vi "Dynamic_call_speed_test.vi"() -> ()   [LabVIEW 2010]
uses:
  Gen Trav/Traverse_cluster.ctl
  Gen Trav/Spacing.ctl
  Controls/Multi_run_mode.ctl
  Globals/Constants_global.vi
panel:
  out "Time taken in seconds":dbl
  out "Error Messages":string
  in  "Traverse line":T1={"Start X"=0.0, "Start Y"=0.0, "Start Z"=0.0, "End X"=0.0, "End Y"=0.0, "End Z"=0.0, "No. of pts."=0, "Spacing"=enum."Linear", "Filename"=path "", "Tunnel Speed"=0.0, "Averaging time (min)"=0.0, "Extra Commands"="", "Specific Arguments"=";2", "Emission Rate (l/min)"=0.0, "Trace Gas Concentration (%)"=0.0, "Density Ratio"="", "Comments"="", "Row No"=0, "Row Type Selector"=enum."Run VI Named:", "Completion time"="", "Row Duration (mins)"=0.0, "No. of Valid pts."=0, "Meas Setup File"=""} {"Row Duration (mins)" format="%#.1f"; "Row No" min=0; "Trace Gas Concentration (%)" min=0.0 format="%#.2f"; "Emission Rate (l/min)" format="%#.2f"; "Tunnel Speed" format="%#.2f"; "Start X" format="%#.2f"; "Start Y" format="%#.2f"; "Start Z" format="%#.2f"; "End X" format="%#.2f"; "End Y" format="%#.2f"; "End Z" format="%#.2f"; "Averaging time (min)" min=0.0 format="%#.1f"}
  in  "Number of calls":i32
  # "X           Y            Z"
  # "Start"
  # "End"
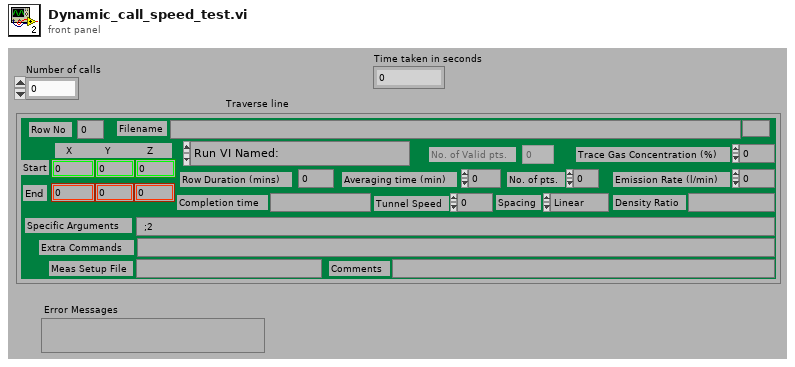
[diagram p1: front panel]
types:
  T1 = typedef "Traverse_cluster.ctl" = cluster{"Start X":dbl, "Start Y":dbl, "Start Z":dbl, "End X":dbl, "End Y":dbl, "End Z":dbl, "No. of pts.":i32, "Spacing":T2, "Filename":path, "Tunnel Speed":dbl, "Averaging time (min)":dbl, "Extra Commands":string, "Specific Arguments":string, "Emission Rate (l/min)":dbl, "Trace Gas Concentration (%)":dbl, "Density Ratio":string, "Comments":string, "Row No":i32, "Row Type Selector":T3, "Completion time":string, "Row Duration (mins)":dbl, "No. of Valid pts.":i32, "Meas Setup File":string}
  T2 = typedef "Spacing.ctl" = enum16{"Linear", "Log", "Gauss", "Specified", "N/A"}
  T3 = typedef "Multi_run_mode.ctl" = enum16{"Move Traverse Only", "Set Tunnel Speed Only", "Set Source Only", "Set Measurement Conditions", "Single Measurement", "Vertical Profile", "Lateral Profile", "Longitudinal Profile", "Explore Volume", "Multi-Axis Profile", "Auto Calibrate", "Meas Fast FID Bkgnd", "Check Beam Power", "Scanning Valve Measurement", "Run VI Named:", "Set ADAM Ch", "Wait (minutes)", "Send Message", "Synchronize With:", "Fall Back to this Row", "Turn Off Row Repeating", "Blank Row"}
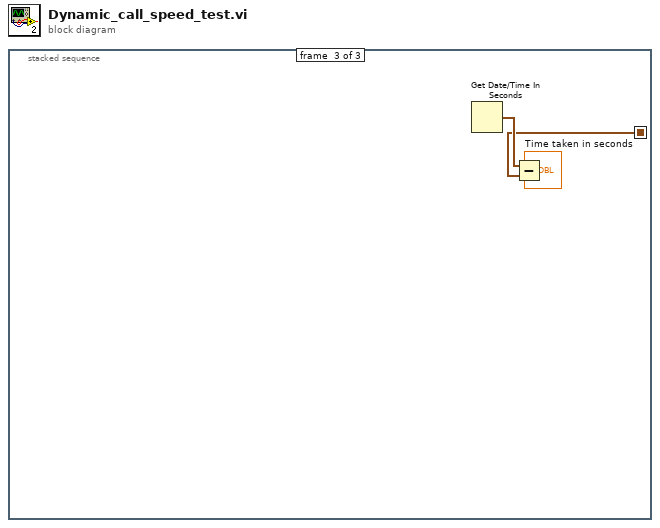
[diagram p0: block diagram]
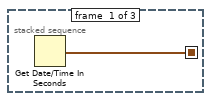
[diagram p2: hidden frame]
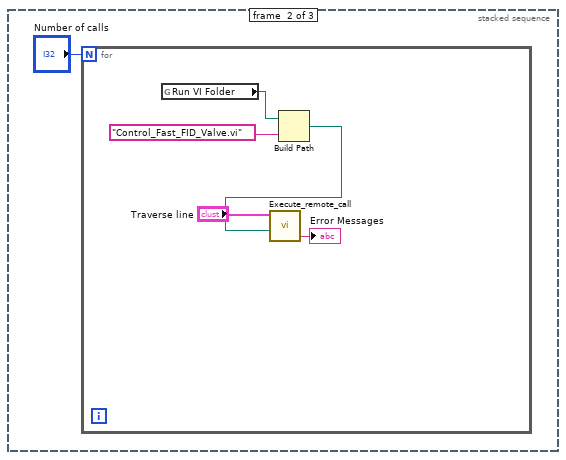
[diagram p3: hidden frame]
diagram:
  n1 = stacked-sequence {
    seq-local: [w1 _ _] -> [_ _ w9]
    frame #0 {
      n2 = Get Date/Time In Seconds() -> (seconds since 1Jan1904=w1:timestamp)
    }
    frame #1 {
      n3 = for {
        N: "Number of calls" -> [_]
        n4 = global read "Constants_global.vi" "Run VI Folder"() -> (w6:path)
        n5 = Build Path(base path=w6, name or relative path="Control_Fast_FID_Valve.vi") -> (appended path=w7:path)
        n6 = call "Execute_remote_call.vi"("Traverse line"="Traverse line", "VI to run"=w7) -> ("Error Messages"=→"Error Messages":string)  [unwired: 4 in, 2 out]
      }
    }
    frame #2 {
      n7 = Get Date/Time In Seconds() -> (seconds since 1Jan1904=w10:timestamp)
      n8 = Subtract(x=w10, y=w9) -> (x-y=→"Time taken in seconds":dbl)
    }
  }
